vi "Client UI.vi"() -> ()   [LabVIEW 2019]
panel:
  out "3D Picture":refnum<vi>(3d-picture)
  in  "Y-Axis":dbl(slide)=1.0 scale=-3.0..3.0
  in  "X-Axis":dbl(slide)=1.0 scale=-3.0..3.0
  in  "Z-Axis":dbl(slide)=1.0 scale=-3.0..3.0
  in  "Enum - Menu":enum16{"Readings", "Manual"}(ring)
  out "Numeric Control":i32
  in  "Stop Button":bool
  # "WIP"
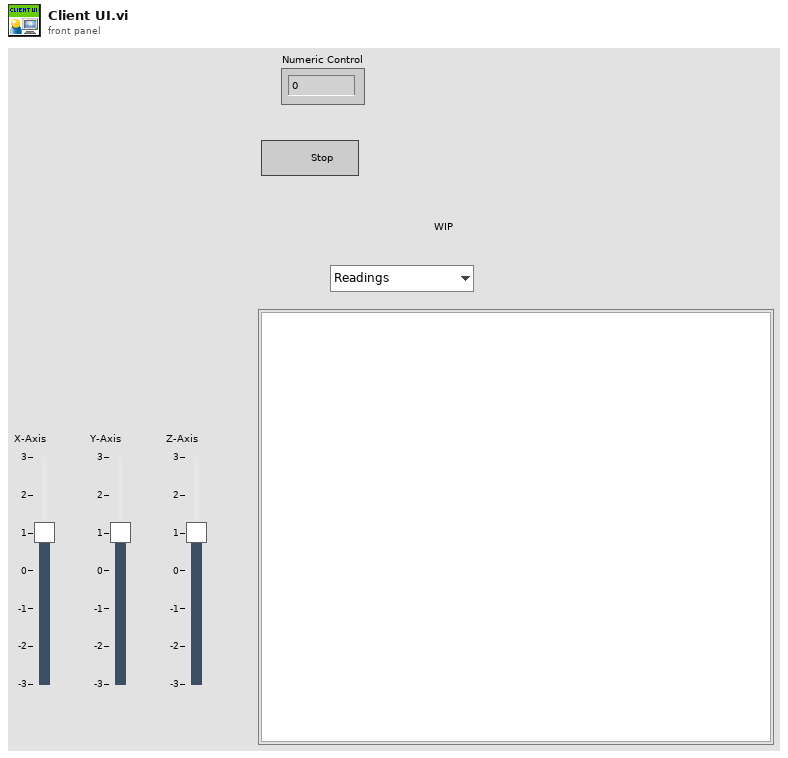
[diagram p1: front panel]
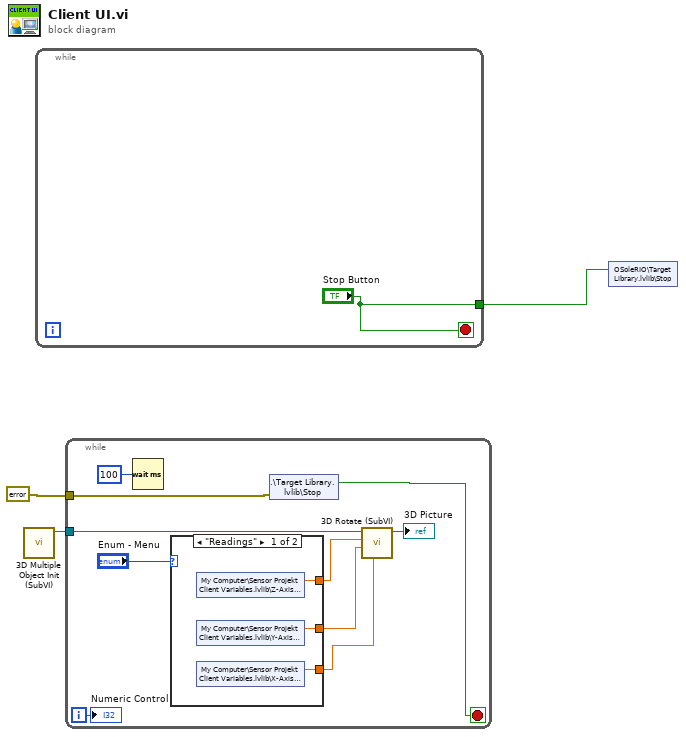
[diagram p0: block diagram]
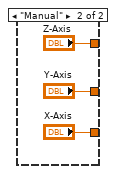
[diagram p2: hidden frame]
diagram:
  n1 = call "3D Multiple Object Init (SubVI).vi"() -> ("SceneObject out"=w2:refnum<vi>)  [unwired: 11 in]
  n2 = while {
    tunnel: ["Stop Button"] -> w3
    stop <- "Stop Button" stop-if-true
  }
  n3 = while {
    tunnel: w2 -> [w10]
    tunnel: errorcluster {"status"=FALSE, "code"=0, "source"=""} ("error in (no error)") -> [w7]
    i -> [w6]
    stop <- w8 stop-if-true
    n4 = Wait (ms)(milliseconds to wait=u32 100) -> ()  [unwired: 1 out]
    n5 = case shown="\"Readings\"" "Enum - Menu" {
      tunnel: [w16 "Y-Axis"] -> w14
      tunnel: [w15 "X-Axis"] -> w13
      tunnel: [w17 "Z-Axis"] -> w5
      frame "Readings" {
        n6 = shared-variable "My Computer\\Sensor Projekt Client Variables.lvlib\\Z-Axis Read"() -> (w17:dbl)  [unwired: 1 in, 1 out]
        n7 = shared-variable "My Computer\\Sensor Projekt Client Variables.lvlib\\Y-Axis Read"() -> (w16:dbl)  [unwired: 1 in, 1 out]
        n8 = shared-variable "My Computer\\Sensor Projekt Client Variables.lvlib\\X-Axis Read"() -> (w15:dbl)  [unwired: 1 in, 1 out]
      }
      frame "Manual" {
      }
    }
    n9 = shared-variable ".\\Target Library.lvlib\\Stop"(error in=w7) -> (w8:bool)  [unwired: 1 out]
    n10 = call "3D Rotate (SubVI).vi"("X-Axis"=w13, "Y-Axis"=w14, "Z-Axis"=w5, "SceneObject in"=w10) -> ("SceneObject out"=→"3D Picture":refnum<vi>)  [unwired: 7 in]
    "Numeric Control" <- w6
  }
  n11 = shared-variable "OSoleRIO\\Target Library.lvlib\\Stop"(w3) -> ()  [unwired: 1 in, 1 out]
